vi "Force Move File.vi"(8 "error in":errorcluster, 10 "Source Path":path, 11 "Target Path in":path) -> (0 "error out":errorcluster, 3 "Target Path out":path)   [LabVIEW 2024]
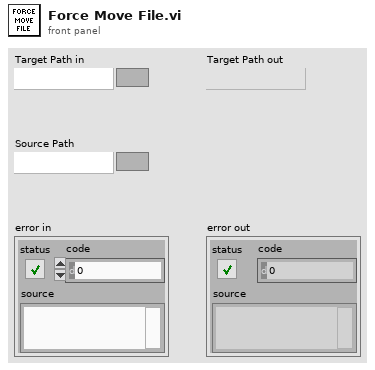
[diagram p1: front panel]
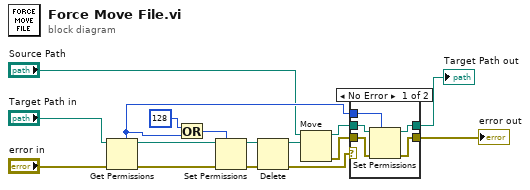
[diagram p0: block diagram]
diagram:
  n1 = Get Permissions(8:"error in", 11:"Target Path in") -> (0:w10:errorcluster, 3:w8:path, 5:w12:i16)  [unwired: 2 out]
  n2 = Or(x=i16 128 ("new permissions"), y=w12) -> (x .or. y?=w11:i16)
  n3 = Set Permissions(7:w11, 8:w10, 11:w8) -> (0:w9:errorcluster, 3:w7:path)  [unwired: 2 in]
  n4 = Delete(path (use dialog)=w7, error in=w9) -> (deleted path=w14:path, error out=w6:errorcluster)  [unwired: 3 in, 1 out]
  n5 = Move(source path="Source Path", 10:w14) -> (error out=w16:errorcluster, 3:w15:path)  [unwired: 3 in, 1 out]
  n6 = case shown="No Error" w6 {
    tunnel: w16 -> [w21 w22]
    tunnel: [w20 w22] -> w3
    tunnel: w15 -> [w19 w23]
    tunnel: w12 -> [w18 _]
    tunnel: [w17 w23] -> w2
    frame No Error {
      n7 = Set Permissions(7:w18, 8:w21, 11:w19) -> (0:w20:errorcluster, 3:w17:path)  [unwired: 2 in]
    }
    frame Error {
    }
  }
  "error out" <- w3
  "Target Path out" <- w2
